vi "how images are displayed.vi"() -> ()   [LabVIEW 2009]
uses:
  <vilib>/picture/picture.llb/Draw True-Color Pixmap.vi
panel:
  out "Mouse Position":cluster{"X":i32, "Y":i32}
  in  "stop":bool
  out "color 2":u32(colorbox)
  out "color":i32 format="%x"
  out "Picture":picture
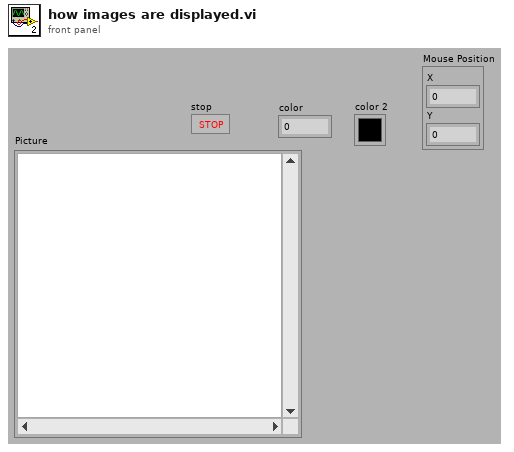
[diagram p1: front panel]
types:
  T1 = typedef "LVMouseTypeDef.ctl" = cluster{"Mouse Position":cluster{"X":i32, "Y":i32}, "Mouse Modifiers":cluster{"Button Down":bool, "Shift Mod":bool, "Menu Mod":bool, "Option Mod":bool}}
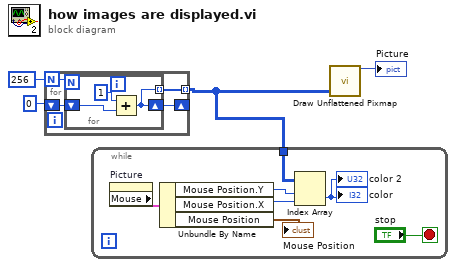
[diagram p0: block diagram]
diagram:
  n1 = for {
    N: 256 -> [w5]
    shift-right: [w7] -> _
    shift-left: 0 -> [w8]
    tunnel: [w6] -> w2 mode=indexing
    n2 = for {
      N: w5 -> [_]
      shift-right: [w10] -> w7
      shift-left: w8 -> [w11]
      tunnel: [w10] -> w6 mode=indexing
      n3 = Add(x=1, y=w11) -> (x+y=w10:i32)
    }
  }
  n4 = while {
    tunnel: w2 -> [w17]
    stop <- "stop" stop-if-true
    n5 = property on="Picture" class="Pict"() -> ("Mouse"=w18:T1)  [unwired: 2 in, 2 out]
    n6 = Unbundle By Name(w18) -> ("Mouse Position.Y"=w12:i32, "Mouse Position.X"=w13:i32, "Mouse Position"=→"Mouse Position":cluster{"X":i32, "Y":i32})
    n7 = Index Array(array=w17, index (row)=w12, index (col)=w13) -> (element=→"color" →"color 2":i32)
  }
  n8 = call-poly <vilib>:"Draw Unflattened Pixmap.vi"("data (RGB format)"=w2) -> ("new picture"=→"Picture":picture)  [unwired: 8 in]
